vi "viLauncher.vi"() -> ()   [LabVIEW 2017]
panel:
  in  "Vi To Launch":path
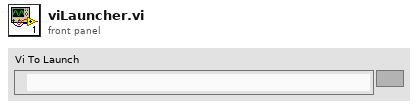
[diagram p1: front panel]
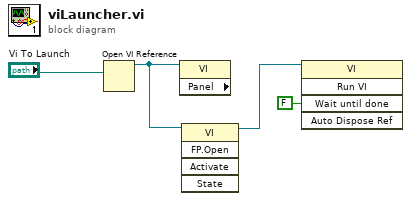
[diagram p0: block diagram]
diagram:
  n1 = Open VI Reference(vi path="Vi To Launch") -> (vi reference=w2:refnum<vi>)  [unwired: 5 in, 1 out]
  n2 = property class="VI" props=["Panel"](reference=w2) -> ()  [unwired: 1 in, 3 out]
  n3 = invoke class="VI" method="FP.Open"(reference=w2) -> (reference out=w1:refnum<vi>)  [unwired: 4 in, 4 out]
  n4 = invoke class="VI" method="Run VI"(reference=w1, "Wait until done"=FALSE ("Wait Until Done")) -> ()  [unwired: 3 in, 5 out]
